vi "DIO.vi"(9 "C O/P":bool[](array[boolean]), 10 "B O/P":bool[](array[boolean]), 11 "A O/P":bool[](array[boolean])) -> (1 "C I/P":bool[](array[boolean]), 2 "B I/P":bool[](array[boolean]), 3 "A I/P":bool[](array[boolean]))   [LabVIEW 2015]
uses:
  <vilib>/rvi/eio/common/nirviEmuTemplateMethod_errors.vi
  <vilib>/eio/EIONode/EIONode.xnode
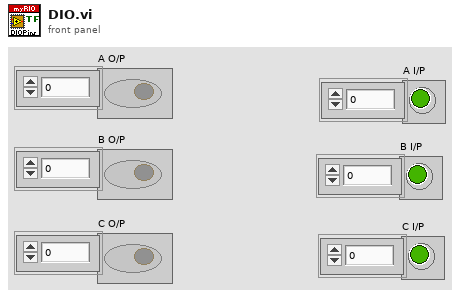
[diagram p1: front panel]
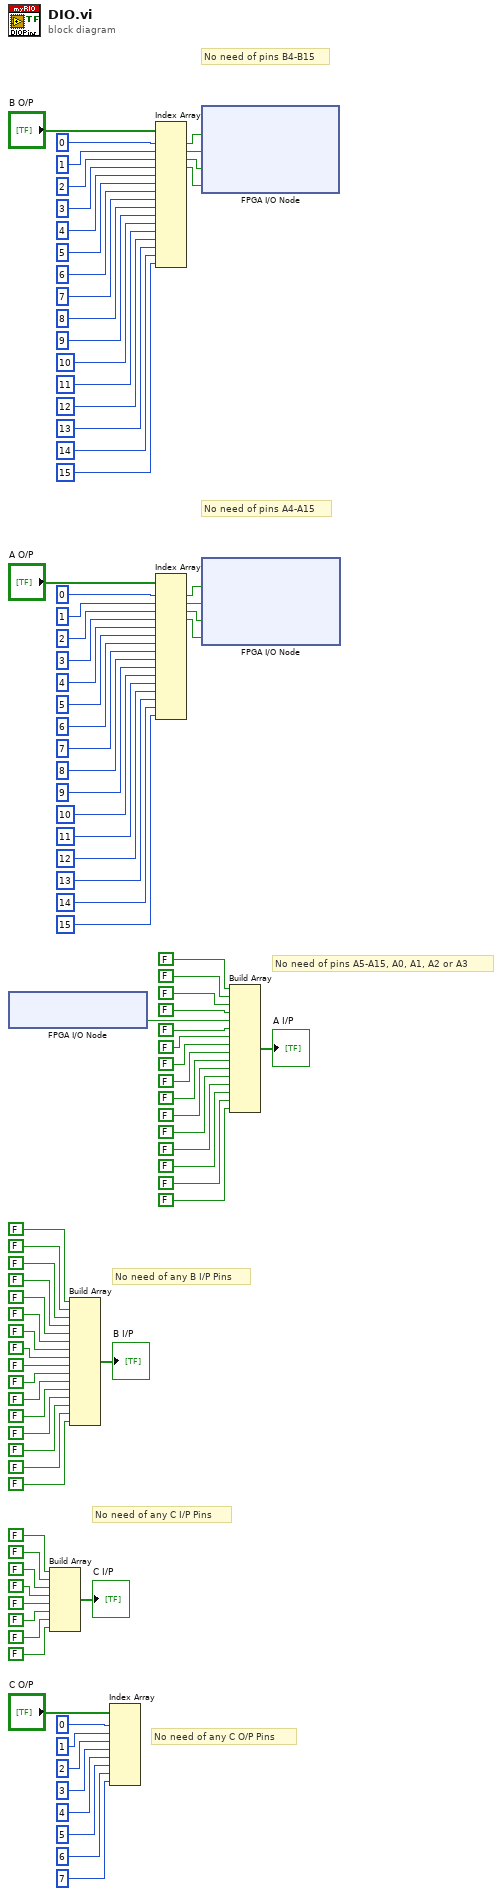
[diagram p0: block diagram]
diagram:
  # "No need of any C O/P Pins"
  # "No need of any C I/P Pins"
  # "No need of any B I/P Pins"
  # "No need of pins A5-A15, A0, A1, A2 or A3"
  # "No need of pins A4-A15"
  # "No need of pins B4-B15"
  n1 = xnode "FPGA I/O Node"() -> ("ConnectorA/DIO4"=w42:bool)  [unwired: 1 in, 1 out]
  n2 = Build Array(FALSE, FALSE ("element"), FALSE ("element"), FALSE ("element"), FALSE ("element"), FALSE ("element"), FALSE ("element"), FALSE ("element")) -> (→"C I/P":bool[])
  n3 = Build Array(FALSE, FALSE ("element"), FALSE ("element"), FALSE ("element"), FALSE ("element"), FALSE ("element"), FALSE ("element"), FALSE ("element"), FALSE ("element"), FALSE ("element"), FALSE ("element"), FALSE ("element"), FALSE ("element"), FALSE ("element"), FALSE ("element"), FALSE ("element")) -> (→"B I/P":bool[])
  n4 = Index Array(array="C O/P", index #1=i16 0, index #2=i16 1, index #3=i16 2, index #4=i16 3, index #5=i16 4, index #6=i16 5, index #7=i16 6, index #8=i16 7) -> ()  [unwired: 8 out]
  n5 = Index Array(array="B O/P", index #1=i16 0, index #2=i16 1, index #3=i16 2, index #4=i16 3, index #5=i16 4, index #6=i16 5, index #7=i16 6, index #8=i16 7, index #9=i16 8, index #10=i16 9, index #11=i16 10, index #12=i16 11, index #13=i16 12, index #14=i16 13, index #15=i16 14, index #16=i16 15) -> (element #1=w47:bool, element #2=w46:bool, element #3=w45:bool, element #4=w44:bool)  [unwired: 12 out]
  n6 = Index Array(array="A O/P", index #1=i16 0, index #2=i16 1, index #3=i16 2, index #4=i16 3, index #5=i16 4, index #6=i16 5, index #7=i16 6, index #8=i16 7, index #9=i16 8, index #10=i16 9, index #11=i16 10, index #12=i16 11, index #13=i16 12, index #14=i16 13, index #15=i16 14, index #16=i16 15) -> (element #1=w92:bool, element #2=w91:bool, element #3=w90:bool, element #4=w89:bool)  [unwired: 12 out]
  n7 = xnode "FPGA I/O Node"("ConnectorB/DIO0"=w47, "ConnectorB/DIO1"=w46, "ConnectorB/DIO2"=w45, "ConnectorB/DIO3"=w44) -> ()  [unwired: 4 in, 4 out]
  n8 = xnode "FPGA I/O Node"("ConnectorA/DIO0"=w92, "ConnectorA/DIO1"=w91, "ConnectorA/DIO2"=w90, "ConnectorA/DIO3"=w89) -> ()  [unwired: 4 in, 4 out]
  n9 = Build Array(FALSE ("element"), FALSE ("element"), FALSE ("element"), FALSE ("element"), w42, FALSE ("element"), FALSE ("element"), FALSE ("element"), FALSE ("element"), FALSE ("element"), FALSE ("element"), FALSE ("element"), FALSE ("element"), FALSE ("element"), FALSE ("element"), FALSE ("element")) -> (→"A I/P":bool[])
